vi "G4SubTemplate_Simple_5x6x5_New.vi"(0 "reference in":refnum<class "G4SubTemplate_Simple_5x6x5.lvclass">, 1 "CreateMethod(Create or look up existing)":T1(ring), 5 "Object name":string, 11 "error in (no error)":errorcluster) -> (4 "reference out":refnum<class "G4SubTemplate_Simple_5x6x5.lvclass">, 6 "NewObjectCreated":bool, 10 "DVRRefOut":refnum<data-value>, 15 "error out":errorcluster)   [LabVIEW 2014, in "G4SubTemplate_Simple_5x6x5.lvclass"]
uses:
  <resource>/Framework/Providers/Open_GDS/ClassProviders/Provider_EndevoGOOP400/Templates/G4SubTemplate_Simple_5x6x5/G4SubTemplate_Simple_5x6x5.lvclass
  <resource>/Framework/Providers/Open_GDS/ClassProviders/Provider_EndevoGOOP400/Templates/G4SubTemplate_Simple_5x6x5/protected/ObjectAttributes.ctl
  <resource>/Framework/Providers/Open_GDS/ClassProviders/Provider_EndevoGOOP400/Templates/G4SubTemplate_Simple_5x6x5/G4SubTemplate_Simple_5x6x5.lvclass/G4SubTemplate_Simple_5x6x5.ctl
  <resource>/Framework/Providers/Open_GDS/ClassProviders/Provider_EndevoGOOP400/Templates/G4BaseTemplate_Simple_5x6x5/G4BaseTemplate_Simple_5x6x5.lvclass
panel:
  in  "DVRRef(Hidden)":refnum<data-value>
  in  "Data":T2 {"Attribute1" format="%.2f"}
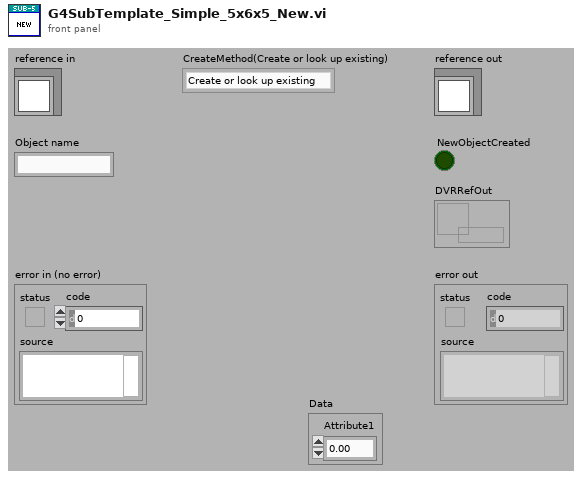
[diagram p1: front panel]
types:
  T1 = enum16{"Create or look up existing", "Look up existing"}
  T2 = typedef "G4SubTemplate_Simple_5x6x5.lvclass/ObjectAttributes.ctl" = cluster{"Attribute1":dbl}
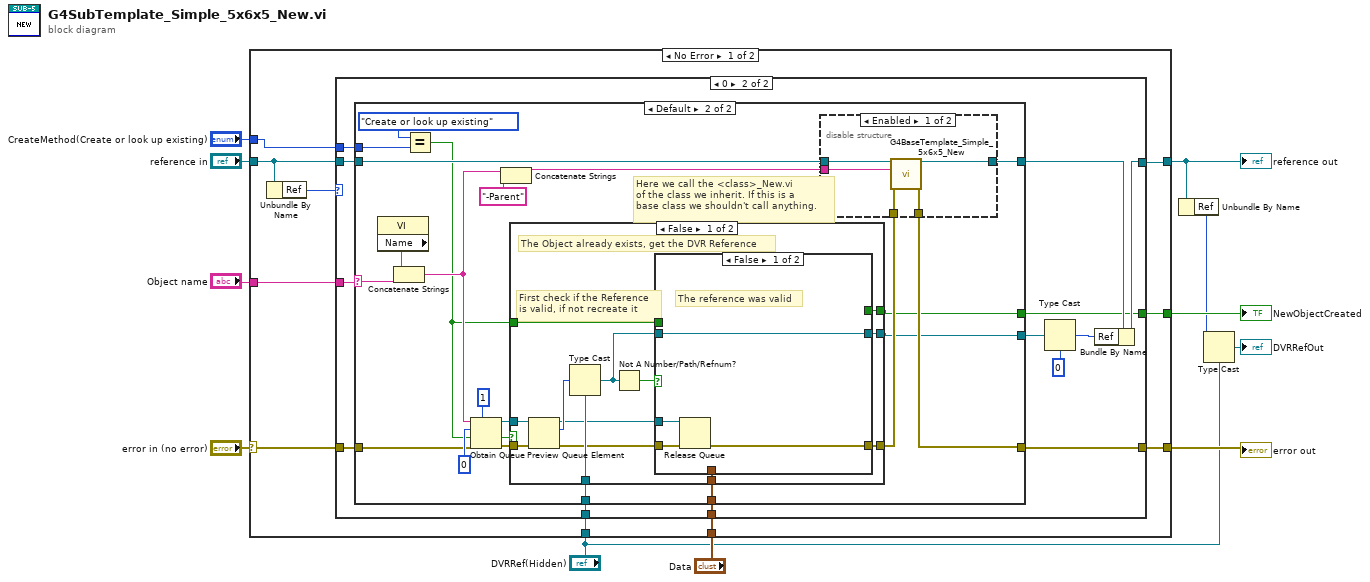
[diagram p0: block diagram]
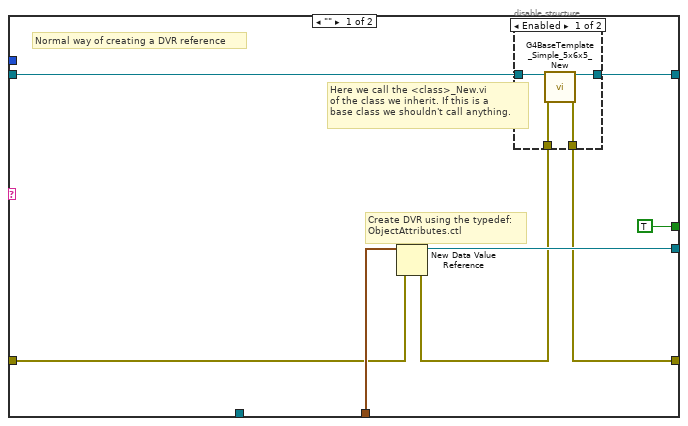
[diagram p3: hidden frame]
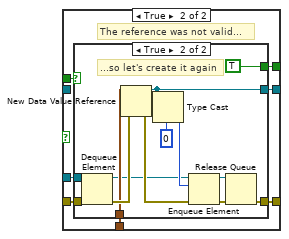
[diagram p5: hidden frame]
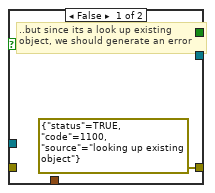
[diagram p6: hidden frame]
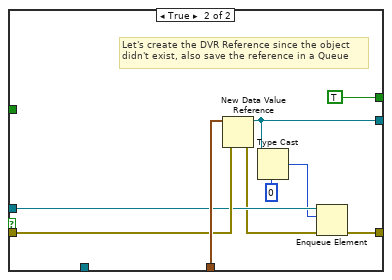
[diagram p7: hidden frame]
diagram:
  n1 = case shown="No Error" "error in (no error)" {
    selector: "error in (no error)" -> [w21 w128]
    tunnel: [w18 w128] -> w7
    tunnel: "CreateMethod(Create or look up existing)" -> [w19 _]
    tunnel: "Object name" -> [w20 _]
    tunnel: "Data" -> [w17 _]
    tunnel: "DVRRef(Hidden)" -> [w16 _]
    tunnel: "reference in" -> [w15 w127]
    tunnel: [w14 w127] -> w4
    tunnel: [w13 _] -> w5
    frame No Error {
      n2 = Unbundle By Name(w15) -> ("Ref"=w12:u32)
      n3 = case shown="0" w12 {
        tunnel: w21 -> [w23 w36]
        tunnel: w20 -> [_ w35]
        tunnel: w19 -> [_ w34]
        tunnel: [w23 w33] -> w18
        tunnel: w17 -> [_ w32]
        tunnel: w15 -> [w22 w30]
        tunnel: [w22 w31] -> w14
        tunnel: w16 -> [_ w28]
        tunnel: [_ w27] -> w13
        frame Default {
          # "The DVR reference has already been created, from this child class's <Child>_New.vi"
        }
        frame 0 {
          n4 = case shown="Default" w35 {
            selector: w35 -> [_ w64]
            tunnel: w36 -> [w43 w61]
            tunnel: [w38 w62] -> w33
            tunnel: w34 -> [_ w71]
            tunnel: w32 -> [w44 w59]
            tunnel: [w42 w53] -> w25
            tunnel: w30 -> [w41 w70]
            tunnel: [w40 w69] -> w29
            tunnel: w28 -> [_ w60]
            tunnel: [TRUE w52] -> w27
            frame "" {
              # "Create DVR using the typedef:\nObjectAttributes.ctl"
              # "Here we call the <class>_New.vi\nof the class we inherit. If this is a\nbase class we shouldn't call anything."
              # "Normal way of creating a DVR reference"
              n5 = New Data Value Reference(data value=w44, error in=w43) -> (data value reference=w42:refnum<data-value>, error out=w39:errorcluster)
              n6 = disable-structure shown="Enabled" {
                disable-tunnel: w41 -> [w48 w50]
                disable-tunnel: [w47 w50] -> w40
                disable-tunnel: w39 -> [w46 w49]
                disable-tunnel: [w45 w49] -> w38
                frame Enabled {
                  n7 = call <resource>:"G4BaseTemplate_Simple_5x6x5_New.vi"("reference in"=w48, "error in (no error)"=w46) -> ("reference out"=w47:refnum<class "G4SubTemplate_Simple_5x6x5.lvclass">, "error out"=w45:errorcluster)  [unwired: 10 in, 2 out]
                }
                frame Disabled {
                }
              }
            }
            frame Default {
              # "Here we call the <class>_New.vi\nof the class we inherit. If this is a\nbase class we shouldn't call anything."
              n8 = property class="VI"() -> ("Name"=w65:string)  [unwired: 2 in, 2 out]
              n9 = Concatenate Strings(w65, w64) -> (w63:string)
              n10 = Equal?(x=T1."Create or look up existing", y=w71) -> (x = y?=w55:bool)
              n11 = Obtain Queue(max queue size (-1, unlimited)=1, name (unnamed)=w63, element data type=u32 0 ("DataRef"), create if not found? (T)=w55, error in (no error)=w61) -> (queue out=w56:refnum<queue>, created new?=w57:bool, error out=w58:errorcluster)
              n12 = Concatenate Strings(w63, "-Parent" ("string")) -> (w66:string)
              n13 = case shown="False" w57 {
                tunnel: w58 -> [w84 w118]
                tunnel: w59 -> [w75 w119]
                tunnel: w56 -> [w85 w117]
                tunnel: [w79 w114] -> w54
                tunnel: [w77 w113] -> w53
                tunnel: w60 -> [w82 _]
                tunnel: [w74 TRUE] -> w52
                tunnel: w55 -> [w73 _]
                frame False {
                  # "First check if the Reference\nis valid, if not recreate it"
                  # "The Object already exists, get the DVR Reference"
                  n14 = Preview Queue Element(queue=w85, error in (no error)=w84) -> (queue out=w76:refnum<queue>, element=w83:u32, error out=w81:errorcluster)  [unwired: 1 in, 1 out]
                  n15 = Type Cast(type=w82, x=w83) -> (*(type *) &x=w78:refnum<data-value>)
                  n16 = Not A Number/Path/Refnum?(number/path/refnum=w78) -> (NaN/Path/Refnum?=w80:bool)
                  n17 = case shown="False" w80 {
                    tunnel: w81 -> [w87 w95]
                    tunnel: [w86 w92] -> w79
                    tunnel: w78 -> [w89 _]
                    tunnel: [w89 w93] -> w77
                    tunnel: w76 -> [w88 w96]
                    tunnel: w75 -> [_ w94]
                    tunnel: [_ w91] -> w74
                    tunnel: w73 -> [_ w90]
                    frame False {
                      # "The reference was valid"
                      n18 = Release Queue(queue=w88, error in (no error)=w87) -> (error out=w86:errorcluster)  [unwired: 1 in, 2 out]
                    }
                    frame True {
                      # "The reference was not valid..."
                      n19 = case shown="True" w90 {
                        tunnel: w96 -> [_ w110]
                        tunnel: w95 -> [_ w109]
                        tunnel: w94 -> [_ w105]
                        tunnel: [_ w102] -> w93
                        tunnel: [errorcluster {"status"=TRUE, "code"=1100, "source"="looking up existing object"} ("error out") w98] -> w92
                        tunnel: [_ TRUE] -> w91
                        frame False {
                          # "..but since its a look up existing\nobject, we should generate an error"
                        }
                        frame True {
                          # "...so let's create it again"
                          n20 = Dequeue Element(queue=w110, error in (no error)=w109) -> (queue out=w103:refnum<queue>, error out=w106:errorcluster)  [unwired: 1 in, 2 out]
                          n21 = New Data Value Reference(data value=w105, error in=w106) -> (data value reference=w102:refnum<data-value>, error out=w104:errorcluster)
                          n22 = Type Cast(type=u32 0 ("ObjectQueue"), x=w102) -> (*(type *) &x=w107:u32)
                          n23 = Enqueue Element(queue=w103, element=w107, error in (no error)=w104) -> (queue out=w99:refnum<queue>, error out=w100:errorcluster)  [unwired: 1 in, 1 out]
                          n24 = Release Queue(queue=w99, error in (no error)=w100) -> (error out=w98:errorcluster)  [unwired: 1 in, 2 out]
                        }
                      }
                    }
                  }
                }
                frame True {
                  # "Let's create the DVR Reference since the object\ndidn't exist, also save the reference in a Queue"
                  n25 = New Data Value Reference(data value=w119, error in=w118) -> (data value reference=w113:refnum<data-value>, error out=w115:errorcluster)
                  n26 = Type Cast(type=u32 0 ("ObjectQueue"), x=w113) -> (*(type *) &x=w112:u32)
                  n27 = Enqueue Element(queue=w117, element=w112, error in (no error)=w115) -> (error out=w114:errorcluster)  [unwired: 1 in, 2 out]
                }
              }
              n28 = disable-structure shown="Enabled" {
                disable-tunnel: w70 -> [w124 w126]
                disable-tunnel: [w123 w126] -> w69
                disable-tunnel: w66 -> [w122 _]
                disable-tunnel: w54 -> [w121 w125]
                disable-tunnel: [w120 w125] -> w62
                frame Enabled {
                  n29 = call <resource>:"G4BaseTemplate_Simple_5x6x5_New.vi"("reference in"=w124, "Object name"=w122, "error in (no error)"=w121) -> ("reference out"=w123:refnum<class "G4SubTemplate_Simple_5x6x5.lvclass">, "error out"=w120:errorcluster)  [unwired: 9 in, 2 out]
                }
                frame Disabled {
                }
              }
            }
          }
          n30 = Type Cast(type=u32 0 ("DataRef"), x=w25) -> (*(type *) &x=w24:u32)
          n31 = Bundle By Name(cluster=w29, "Ref"=w24) -> (w31:refnum<class "G4SubTemplate_Simple_5x6x5.lvclass">)
        }
      }
    }
    frame Error {
    }
  }
  "error out" <- w7
  "reference out" <- w4
  "NewObjectCreated" <- w5
  n32 = Unbundle By Name(w4) -> ("Ref"=w3:u32)
  n33 = Type Cast(type="DVRRef(Hidden)", x=w3) -> (*(type *) &x=→"DVRRefOut":refnum<data-value>)
